vi "rsidr_core_global.vi"() -> ()   [LabVIEW 2020, in "Rohde&Schwarz RTx Oscilloscopes.lvlib"] (continued)
modulation.\n\nAvailable Repeated Capabilities:\nNone\n\nRemote-control command(s):\nWGENerator:MODulation:ASK:FREQuency"}, {"Level"=5, "Class Only"=FALSE, "Identifier"="RSRTX_ATTR_WAVEFORM_GENERATOR_ASK_MODULATION_DEPTH", "Descriptive Name"="Waveform Generator ASK Modulation Depth", "Data Type"=1, "Command"="WGEN:MOD:ASK:DEPT", "Access"=2, "Range Table"="", "Read Callback"="", "Write Callback"="", "Supported Models"="", "Instrument Options"="", "Flags"=0, "Help"="Sets the ASK modulation depth.\n\nAvailable Repeated Capabilities:\nNone\n\nRemote-control command(s):\nWGENerator:MODulation:ASK:DEPTh"}, {"Level"=4, "Class Only"=TRUE, "Identifier"="", "Descriptive Name"="FSK", "Data Type"=0, "Command"="", "Access"=0, "Range Table"="", "Read Callback"="", "Write Callback"="", "Supported Models"="", "Instrument Options"="", "Flags"=0, "Help"="For frequency shift keying (FSK) modulation, the signal switches between Frequency 1 and Frequency 2 at a Hop rate."}, {"Level"=5, "Class Only"=FALSE, "Identifier"="RSRTX_ATTR_WAVEFORM_GENERATOR_FSK_MODULATION_HOPPING_FREQUENCY", "Descriptive Name"="Waveform Generator FSK Modulation Hopping Frequency", "Data Type"=1, "Command"="WGEN:MOD:FSK:HFRE", "Access"=2, "Range Table"="", "Read Callback"="", "Write Callback"="", "Supported Models"="", "Instrument Options"="", "Flags"=0, "Help"="Sets the hopping frequency.\n\nAvailable Repeated Capabilities:\nNone\n\nRemote-control command(s):\nWGENerator:MODulation:FSK:HFREquency"}, {"Level"=5, "Class Only"=FALSE, "Identifier"="RSRTX_ATTR_WAVEFORM_GENERATOR_FSK_MODULATION_RATE", "Descriptive Name"="Waveform Generator FSK Modulation Rate", "Data Type"=1, "Command"="WGEN:MOD:FSK:RATE", "Access"=2, "Range Table"="", "Read Callback"="", "Write Callback"="", "Supported Models"="", "Instrument Options"="", "Flags"=0, "Help"="Sets the hop rate, the time before a switch from the carrier frequency and the modulation frequency.\n\nAvailable Repeated Capabilities:\nNone\n\nRemote-control command(s):\nWGENerator:MODulation:FSK:RATE"}, {"Level"=3, "Class Only"=TRUE, "Identifier"="", "Descriptive Name"="Sweep", "Data Type"=0, "Command"="", "Access"=0, "Range Table"="", "Read Callback"="", "Write Callback"="", "Supported Models"="", "Instrument Options"="", "Flags"=0, "Help"="In the sweep mode, the R&S RTO generates a signal whose frequency gradually changes from the Start frequency to the Stop freuqency for a certain Sweep time."}, {"Level"=4, "Class Only"=FALSE, "Identifier"="RSRTX_ATTR_WAVEFORM_GENERATOR_SWEEP_ENABLED", "Descriptive Name"="Waveform Generator Sweep Enabled", "Data Type"=3, "Command"="WGEN:SWE", "Access"=2, "Range Table"="", "Read Callback"="", "Write Callback"="", "Supported Models"="", "Instrument Options"="", "Flags"=0, "Help"="Enables the sweep.\n\nAvailable Repeated Capabilities:\nNone\n\nRemote-control command(s):\nWGENerator:SWEep[:ENABle]"}, {"Level"=4, "Class Only"=FALSE, "Identifier"="RSRTX_ATTR_WAVEFORM_GENERATOR_SWEEP_TYPE", "Descriptive Name"="Waveform Generator Sweep Type", "Data Type"=0, "Command"="WGEN:SWE:TYPE", "Access"=2, "Range Table"="rsrtx_rngWaveformGeneratorSweepType", "Read Callback"="", "Write Callback"="", "Supported Models"="", "Instrument Options"="", "Flags"=0, "Help"="Configures the sweep type.\n\nAvailable Repeated Capabilities:\nNone\n\nRemote-control command(s):\nWGENerator:SWEep:TYPE"}, {"Level"=4, "Class Only"=FALSE, "Identifier"="RSRTX_ATTR_WAVEFORM_GENERATOR_SWEEP_START_FREQUENCY", "Descriptive Name"="Waveform Generator Sweep Start Frequency", "Data Type"=1, "Command"="WGEN:SWE:FST", "Access"=2, "Range Table"="", "Read Callback"="", "Write Callback"="", "Supported Models"="", "Instrument Options"="", "Flags"=0, "Help"="Sets the start frequency of the sweep range.\n\nAvailable Repeated Capabilities:\nNone\n\nRemote-control command(s):\nWGENerator:SWEep:FSTart"}, {"Level"=4, "Class Only"=FALSE, "Identifier"="RSRTX_ATTR_WAVEFORM_GENERATOR_SWEEP_STOP_FREQUENCY", "Descriptive Name"="Waveform Generator Sweep Stop Frequency", "Data Type"=1, "Command"="WGEN:SWE:FEND", "Access"=2, "Range Table"="", "Read Callback"="", "Write Callback"="", "Supported Models"="", "Instrument Options"="", "Flags"=0, "Help"="Sets the stop frequency of the sweep range.\n\nAvailable Repeated Capabilities:\nNone\n\nRemote-control command(s):\nWGENerator:SWEep:FEND"}, {"Level"=4, "Class Only"=FALSE, "Identifier"="RSRTX_ATTR_WAVEFORM_GENERATOR_SWEEP_TIME", "Descriptive Name"="Waveform Generator Sweep Time", "Data Type"=1, "Command"="WGEN:SWE:TIME", "Access"=2, "Range Table"="", "Read Callback"="", "Write Callback"="", "Supported Models"="", "Instrument Options"="", "Flags"=0, "Help"="Sets the duration of the sweep.\n\nAvailable Repeated Capabilities:\nNone\n\nRemote-control command(s):\nWGENerator:SWEep:TIME"}, {"Level"=3, "Class Only"=TRUE, "Identifier"="", "Descriptive Name"="Arbitrary", "Data Type"=0, "Command"="", "Access"=0, "Range Table"="", "Read Callback"="", "Write Callback"="", "Supported Models"="", "Instrument Options"="", "Flags"=0, "Help"="The arbitrary waveform generator allows you to output a user-defined waveform for testing your devices. You can output a waveform from a file or from the current R&S RTO reference curve format. Files in *.csv and *.bin formats are supported. This files must follow a defined structure."}, {"Level"=4, "Class Only"=FALSE, "Identifier"="RSRTX_ATTR_WAVEFORM_GENERATOR_ARBITRARY_FILE_NAME", "Descriptive Name"="Waveform Generator Arbitrary File Name", "Data Type"=2, "Command"="WGEN:ARB:NAME", "Access"=2, "Range Table"="", "Read Callback"="", "Write Callback"="", "Supported Models"="", "Instrument Options"="", "Flags"=0, "Help"="Sets the file path and the file for an arbitrary waveform.\n\nAvailable Repeated Capabilities:\nNone\n\nRemote-control command(s):\nWGENerator:ARBitrary[:FILE]:NAME"}, {"Level"=4, "Class Only"=FALSE, "Identifier"="RSRTX_ATTR_WAVEFORM_GENERATOR_ARBITRARY_OPEN_FILE", "Descriptive Name"="Waveform Generator Arbitrary Open File", "Data Type"=4, "Command"="WGEN:ARB:OPEN", "Access"=1, "Range Table"="", "Read Callback"="", "Write Callback"="", "Supported Models"="", "Instrument Options"="", "Flags"=0, "Help"="Loads the arbitrary waveform.\n\nAvailable Repeated Capabilities:\nNone\n\nRemote-control command(s):\nWGENerator:ARBitrary[:FILE]:OPEN"}, {"Level"=4, "Class Only"=FALSE, "Identifier"="RSRTX_ATTR_WAVEFORM_GENERATOR_ARBITRARY_SOURCE", "Descriptive Name"="Waveform Generator Arbitrary Source", "Data Type"=0, "Command"="WGEN:ARB:SOUR", "Access"=2, "Range Table"="RsRtx_rngWaveformGeneratorArbitrarySource", "Read Callback"="", "Write Callback"="", "Supported Models"="", "Instrument Options"="", "Flags"=0, "Help"="Selects the oscilloscope source, from which the arbitrary signal is loaded.\n\nAvailable Repeated Capabilities:\nNone\n\nRemote-control command(s):\nWGENerator:ARBitrary:SOURce"}, {"Level"=4, "Class Only"=FALSE, "Identifier"="RSRTX_ATTR_WAVEFORM_GENERATOR_ARBITRARY_UPDATE", "Descriptive Name"="Waveform Generator Arbitrary Update", "Data Type"=4, "Command"="WGEN:ARB:UPD", "Access"=1, "Range Table"="", "Read Callback"="", "Write Callback"="", "Supported Models"="", "Instrument Options"="", "Flags"=0, "Help"="Loads the waveform from the selected signal source.\n\nAvailable Repeated Capabilities:\nNone\n\nRemote-control command(s):\nWGENerator:ARBitrary:UPDate"}, {"Level"=4, "Class Only"=FALSE, "Identifier"="RSRTX_ATTR_WAVEFORM_GENERATOR_ARBITRARY_RANGE_START", "Descriptive Name"="Waveform Generator Arbitrary Range Start", "Data Type"=1, "Command"="WGEN:ARB:RANG:START", "Access"=2, "Range Table"="", "Read Callback"="", "Write Callback"="", "Supported Models"="", "Instrument Options"="", "Flags"=0, "Help"="Sets the start time of the copied waveform part in seconds.\n\nAvailable Repeated Capabilities:\nNone\n\nRemote-control command(s):\nWGENerator:ARBitrary:RANGe:START"}, {"Level"=4, "Class Only"=FALSE, "Identifier"="RSRTX_ATTR_WAVEFORM_GENERATOR_ARBITRARY_RANGE_END", "Descriptive Name"="Waveform Generator Arbitrary Range End", "Data Type"=1, "Command"="WGEN:ARB:RANG:STOP", "Access"=2, "Range Table"="", "Read Callback"="", "Write Callback"="", "Supported Models"="", "Instrument Options"="", "Flags"=0, "Help"="Sets the end time of the copied waveform part in seconds.\n\nAvailable Repeated Capabilities:\nNone\n\nRemote-control command(s):\nWGENerator:ARBitrary:RANGe:STOP"}, {"Level"=4, "Class Only"=FALSE, "Identifier"="RSRTX_ATTR_WAVEFORM_GENERATOR_ARBITRARY_DISPLAY_ENABLE", "Descriptive Name"="Waveform Generator Arbitrary Display Enable", "Data Type"=3, "Command"="WGEN:ARB:VIS", "Access"=2, "Range Table"="", "Read Callback"="", "Write Callback"="", "Supported Models"="", "Instrument Options"="", "Flags"=0, "Help"="Enables the display of the arbitrary waveform.\n\nAvailable Repeated Capabilities:\nNone\n\nRemote-control command(s):\nWGENerator:ARBitrary:VISible"}, {"Level"=3, "Class Only"=TRUE, "Identifier"="", "Descriptive Name"="Output", "Data Type"=0, "Command"="", "Access"=0, "Range Table"="", "Read Callback"="", "Write Callback"="", "Supported Models"="", "Instrument Options"="", "Flags"=0, "Help"="Configures the output values of generator."}, {"Level"=4, "Class Only"=FALSE, "Identifier"="RSRTX_ATTR_WAVEFORM_GENERATOR_OUTPUT_ENABLED", "Descriptive Name"="Waveform Generator Output Enabled", "Data Type"=3, "Command"="WGEN:OUTP", "Access"=2, "Range Table"="", "Read Callback"="", "Write Callback"="", "Supported Models"="", "Instrument Options"="", "Flags"=0, "Help"="Enables the waveform generator and outputs the waveform.\n\nAvailable Repeated Capabilities:\nNone\n\nRemote-control command(s):\nWGENerator:OUTPut[:ENABle]"}, {"Level"=4, "Class Only"=FALSE, "Identifier"="RSRTX_ATTR_WAVEFORM_GENERATOR_OUTPUT_AMPLITUDE", "Descriptive Name"="Waveform Generator Output Amplitude", "Data Type"=1, "Command"="WGEN:VOLT", "Access"=2, "Range Table"="", "Read Callback"="", "Write Callback"="", "Supported Models"="", "Instrument Options"="", "Flags"=0, "Help"="Sets the amplitude, peak to peak voltage, of the output waveform. This is defined as the voltage difference between the maximum and the minimum voltage levels.\n\nAvailable Repeated Capabilities:\nNone\n\nRemote-control command(s):\nWGENerator:VOLTage"}, {"Level"=4, "Class Only"=FALSE, "Identifier"="RSRTX_ATTR_WAVEFORM_GENERATOR_OUTPUT_OFFSET", "Descriptive Name"="Waveform Generator Output Offset", "Data Type"=1, "Command"="WGEN:VOLT:OFFS", "Access"=2, "Range Table"="", "Read Callback"="", "Write Callback"="", "Supported Models"="", "Instrument Options"="", "Flags"=0, "Help"="Sets a voltage offset.\n\nAvailable Repeated Capabilities:\nNone\n\nRemote-control command(s):\nWGENerator:VOLTage:OFFSet"}, {"Level"=4, "Class Only"=FALSE, "Identifier"="RSRTX_ATTR_WAVEFORM_GENERATOR_OUTPUT_USER_LOAD", "Descriptive Name"="Waveform Generator Output User Load", "Data Type"=0, "Command"="WGEN:OUTP:LOAD", "Access"=2, "Range Table"="RsRtx_rngWaveformGeneratorLoad", "Read Callback"="", "Write Callback"="", "Supported Models"="", "Instrument Options"="", "Flags"=0, "Help"="Sets the load of the DUT at its connection.\n\nAvailable Repeated Capabilities:\nNone\n\nRemote-control command(s):\nWGENerator:OUTPut:LOAD"}, {"Level"=4, "Class Only"=FALSE, "Identifier"="RSRTX_ATTR_WAVEFORM_GENERATOR_OUTPUT_DESTINATION", "Descriptive Name"="Waveform Generator Output Destination", "Data Type"=0, "Command"="WGEN:OUTP:DEST", "Access"=2, "Range Table"="RsRtx_rngWaveformGeneratorOutputDestination", "Read Callback"="", "Write Callback"="", "Supported Models"="", "Instrument Options"="", "Flags"=0, "Help"="Configures the output destination.\n\nAvailable Repeated Capabilities:\nNone\n\nRemote-control command(s):\nWGENerator:OUTPut:DESTination"}, {"Level"=3, "Class Only"=TRUE, "Identifier"="", "Descriptive Name"="Noise", "Data Type"=0, "Command"="", "Access"=0, "Range Table"="", "Read Callback"="", "Write Callback"="", "Supported Models"="", "Instrument Options"="", "Flags"=0, "Help"="Configures the noise of attributes."}, {"Level"=4, "Class Only"=FALSE, "Identifier"="RSRTX_ATTR_WAVEFORM_GENERATOR_NOISE_LEVEL_PERCENT", "Descriptive Name"="Waveform Generator Noise Level Percent", "Data Type"=1, "Command"="WGEN:NOIS:REL", "Access"=2, "Range Table"="RsRtx_rngPercent", "Read Callback"="", "Write Callback"="", "Supported Models"="", "Instrument Options"="", "Flags"=0, "Help"="Sets the noise level in percentage of the amplitude.\n\nAvailable Repeated Capabilities:\nNone\n\nRemote-control command(s):\nWGENerator:NOISe:RELative"}, {"Level"=4, "Class Only"=FALSE, "Identifier"="RSRTX_ATTR_WAVEFORM_GENERATOR_NOISE_ABSOLUTE_LEVEL", "Descriptive Name"="Waveform Generator Noise Absolute Level", "Data Type"=1, "Command"="WGEN:NOIS:ABS", "Access"=2, "Range Table"="", "Read Callback"="", "Write Callback"="", "Supported Models"="", "Instrument Options"="", "Flags"=0, "Help"="Sets the level of the noise in volts.\n\nAvailable Repeated Capabilities:\nNone\n\nRemote-control command(s):\nWGENerator:NOISe:ABSolute"}, {"Level"=3, "Class Only"=TRUE, "Identifier"="", "Descriptive Name"="Burst", "Data Type"=0, "Command"="", "Access"=0, "Range Table"="", "Read Callback"="", "Write Callback"="", "Supported Models"="", "Instrument Options"="", "Flags"=0, "Help"="This class contains settings for the waveform generator burst mode. With the burst mode, you can output a waveform for a set number of times."}, {"Level"=4, "Class Only"=FALSE, "Identifier"="RSRTX_ATTR_WAVEFORM_GENERATOR_BURST_ENABLE", "Descriptive Name"="Waveform Generator Burst Enable", "Data Type"=3, "Command"="WGEN:BURS", "Access"=2, "Range Table"="", "Read Callback"="", "Write Callback"="", "Supported Models"="", "Instrument Options"="", "Flags"=0, "Help"="Enables or disables the burst for the generator.\n\nAvailable Repeated Capabilities:\nNone\n\nRemote-control command(s):\nWGENerator:BURSt[:STATe]"}, {"Level"=4, "Class Only"=FALSE, "Identifier"="RSRTX_ATTR_WAVEFORM_GENERATOR_BURST_CYCLES", "Descriptive Name"="Waveform Generator Burst Cycles", "Data Type"=0, "Command"="WGEN:BURS:NCYC", "Access"=2, "Range Table"="RsRtx_rngBurstCycles", "Read Callback"="", "Write Callback"="", "Supported Models"="", "Instrument Options"="", "Flags"=0, "Help"="Sets the number of times the generator outputs one cycle of the waveform per burst.\n\nAvailable Repeated Capabilities:\nNone\n\nRemote-control command(s):\nWGENerator:BURSt:NCYCle"}, {"Level"=4, "Class Only"=FALSE, "Identifier"="RSRTX_ATTR_WAVEFORM_GENERATOR_BURST_IDLE_TIME", "Descriptive Name"="Waveform Generator Burst Idle Time", "Data Type"=1, "Command"="WGEN:BURS:ITIM", "Access"=2, "Range Table"="RsRtx_rngBurstIdleTime", "Read Callback"="", "Write Callback"="", "Supported Models"="", "Instrument Options"="", "Flags"=0, "Help"="Sets the idle time between two burst cycles.\n\nAvailable Repeated Capabilities:\nNone\n\nRemote-control command(s):\nWGENerator:BURSt:ITIMe"}, {"Level"=4, "Class Only"=FALSE, "Identifier"="RSRTX_ATTR_WAVEFORM_GENERATOR_BURST_PHASE_OFFSET", "Descriptive Name"="Waveform Generator Burst Phase Offset", "Data Type"=1, "Command"="WGEN:BURS:PHAS", "Access"=2, "Range Table"="RsRtx_rng360Degrees", "Read Callback"="", "Write Callback"="", "Supported Models"="", "Instrument Options"="", "Flags"=0, "Help"="Sets the start phase of the burst.\n\nAvailable Repeated Capabilities:\nNone\n\nRemote-control command(s):\nWGENerator:BURSt:PHASe"}, {"Level"=4, "Class Only"=FALSE, "Identifier"="RSRTX_ATTR_WAVEFORM_GENERATOR_BURST_TRIGGER_MODE", "Descriptive Name"="Waveform Generator Burst Trigger Mode", "Data Type"=0, "Command"="WGEN:BURS:TRIG", "Access"=2, "Range Table"="RsRtx_rngBurstTriggerMode", "Read Callback"="", "Write Callback"="", "Supported Models"="", "Instrument Options"="", "Flags"=0, "Help"="Selects the trigger mode. Each time the generator receives a trigger, it outputs a burst with the number of cycles defined with RSRTX_ATTR_WAVEFORM_GENERATOR_BURST_CYCLES.\n\nAvailable Repeated Capabilities:\nNone\n\nRemote-control command(s):\nWGENerator:BURSt:TRIGger[:MODE]"}, {"Level"=4, "Class Only"=FALSE, "Identifier"="RSRTX_ATTR_WAVEFORM_GENERATOR_BURST_TRIGGER_SINGLE", "Descriptive Name"="Waveform Generator Burst Trigger Single", "Data Type"=4, "Command"="WGEN:BURS:TRIG:SING", "Access"=1, "Range Table"="", "Read Callback"="", "Write Callback"="", "Supported Models"="", "Instrument Options"="", "Flags"=0, "Help"="Outputs one burst if RSRTX_ATTR_WAVEFORM_GENERATOR_BURST_TRIGGER_MODE is set to Single.\n\nAvailable Repeated Capabilities:\nNone\n\nRemote-control command(s):\nWGENerator:BURSt:TRIGger:SINGle"}, {"Level"=2, "Class Only"=TRUE, "Identifier"="", "Descriptive Name"="Pattern Generator", "Data Type"=0, "Command"="", "Access"=0, "Range Table"="", "Read Callback"="", "Write Callback"="", "Supported Models"="", "Instrument Options"="", "Flags"=0, "Help"="Includes an integrated pattern generator which can generate patterns during testing."}, {"Level"=3, "Class Only"=FALSE, "Identifier"="RSRTX_ATTR_PATTERN_GENERATOR_ENABLED", "Descriptive Name"="Pattern Generator Enabled", "Data Type"=3, "Command"="PGEN:PATT:STAT", "Access"=2, "Range Table"="", "Read Callback"="", "Write Callback"="", "Supported Models"="", "Instrument Options"="", "Flags"=0, "Help"="Enables the pattern generator and outputs the waveform.\n\nAvailable Repeated Capabilities:\nNone\n\nRemote-control command(s):\nPGENerator:PATTern:STATe"}, {"Level"=3, "Class Only"=FALSE, "Identifier"="RSRTX_ATTR_PATTERN_GENERATOR_FUNCTION_TYPE", "Descriptive Name"="Pattern Generator Function Type", "Data Type"=0, "Command"="PGEN:FUNC", "Access"=2, "Range Table"="RsRtx_rngPatternGeneratorFunctionType", "Read Callback"="", "Write Callback"="", "Supported Models"="", "Instrument Options"="", "Flags"=0, "Help"="Selects the pattern generator function.\n\nAvailable Repeated Capabilities:\nNone\n\nRemote-control command(s):\nPGENerator:FUNCtion"}, {"Level"=3, "Class Only"=FALSE, "Identifier"="RSRTX_ATTR_PATTERN_GENERATOR_FREQUENCY", "Descriptive Name"="Pattern Generator Frequency", "Data Type"=1, "Command"="PGEN:PATT:FREQ", "Access"=2, "Range Table"="", "Read Callback"="", "Write Callback"="", "Supported Models"="", "Instrument Options"="", "Flags"=0, "Help"="Configures generator frequency.\n\nAvailable Repeated Capabilities:\nNone\n\nRemote-control command(s):\nPGENerator:PATTern:FREQuency"}, {"Level"=3, "Class Only"=FALSE, "Identifier"="RSRTX_ATTR_PATTERN_GENERATOR_PERIOD", "Descriptive Name"="Pattern Generator Period", "Data Type"=1, "Command"="PGEN:PATT:PER", "Access"=2, "Range Table"="", "Read Callback"="", "Write Callback"="", "Supported Models"="", "Instrument Options"="", "Flags"=0, "Help"="Configures pattern generator period.\n\nAvailable Repeated Capabilities:\nNone\n\nRemote-control command(s):\nPGENerator:PATTern:PERiod"}, {"Level"=3, "Class Only"=FALSE, "Identifier"="RSRTX_ATTR_PATTERN_GENERATOR_POLARITY", "Descriptive Name"="Pattern Generator Polarity", "Data Type"=0, "Command"="PGEN:PATT:SQU:POL", "Access"=2, "Range Table"="rsrtx_rngChannelPolarity", "Read Callback"="", "Write Callback"="", "Supported Models"="", "Instrument Options"="", "Flags"=0, "Help"="Configures the waveform polarity.\n\nAvailable Repeated Capabilities:\nNone\n\nRemote-control command(s):\nPGENerator:PATTern:SQUarewave:POLarity"}, {"Level"=3, "Class Only"=FALSE, "Identifier"="RSRTX_ATTR_PATTERN_GENERATOR_OUTPUT_VOLTAGE", "Descriptive Name"="Pattern Generator Output Voltage", "Data Type"=1, "Command"="PGEN:OUTP:VOLT", "Access"=2, "Range Table"="", "Read Callback"="", "Write Callback"="", "Supported Models"="", "Instrument Options"="", "Flags"=0, "Help"="Sets the output voltage of the generated pattern signal.\n\nAvailable Repeated Capabilities:\nNone\n\nRemote-control command(s):\nPGENerator:OUTPut:VOLTage"}, {"Level"=3, "Class Only"=FALSE, "Identifier"="RSRTX_ATTR_PATTERN_GENERATOR_DUTY_CYCLE", "Descriptive Name"="Pattern Generator Duty Cycle", "Data Type"=1, "Command"="PGEN:PATT:SQU:DCYC", "Access"=2, "Range Table"="", "Read Callback"="", "Write Callback"="", "Supported Models"="", "Instrument Options"="", "Flags"=0, "Help"="Configures the waveform duty cycle.\n\nAvailable Repeated Capabilities:\nNone\n\nRemote-control command(s):\nPGENerator:PATTern:SQUarewave:DCYCle"}, {"Level"=3, "Class Only"=FALSE, "Identifier"="RSRTX_ATTR_PATTERN_GENERATOR_SAMPLE_TIME", "Descriptive Name"="Pattern Generator Sample Time", "Data Type"=1, "Command"="PGEN:PATT:STIM", "Access"=2, "Range Table"="", "Read Callback"="", "Write Callback"="", "Supported Models"="", "Instrument Options"="", "Flags"=0, "Help"="Configures generator sample time.\n\nAvailable Repeated Capabilities:\nNone\n\nRemote-control command(s):\nPGENerator:PATTern:STIMe"}, {"Level"=3, "Class Only"=FALSE, "Identifier"="RSRTX_ATTR_PATTERN_GENERATOR_COUNTER_DIRECTION", "Descriptive Name"="Pattern Generator Counter Direction", "Data Type"=0, "Command"="PGEN:PATT:COUN:DIR", "Access"=2, "Range Table"="RsRtx_rngPatternGeneratorCounterDirection", "Read Callback"="", "Write Callback"="", "Supported Models"="", "Instrument Options"="", "Flags"=0, "Help"="Configures the counter direction.\n\nAvailable Repeated Capabilities:\nNone\n\nRemote-control command(s):\nPGENerator:PATTern:COUNter:DIRection"}, {"Level"=3, "Class Only"=FALSE, "Identifier"="RSRTX_ATTR_PATTERN_GENERATOR_COUNTER_FREQUENCY", "Descriptive Name"="Pattern Generator Counter Frequency", "Data Type"=1, "Command"="PGEN:PATT:COUN:FREQ", "Access"=2, "Range Table"="", "Read Callback"="", "Write Callback"="", "Supported Models"="", "Instrument Options"="", "Flags"=0, "Help"="Defines the frequency value of the pattern generator counter function. The user frequency always refers to the switching of the pattern condition. This results in square waveforms for individual pins.\n\nPin: Frequency\nS0: f/2\nS1: f/4\nS2: f/8\nS3: f/16\n\nAvailable Repeated Capabilities:\nNone\n\nRemote-control command(s):\nPGENerator:PATTern:COUNter:FREQuency"}, {"Level"=3, "Class Only"=FALSE, "Identifier"="RSRTX_ATTR_PATTERN_GENERATOR_BURST_ENABLED", "Descriptive Name"="Pattern Generator Burst Enabled", "Data Type"=3, "Command"="PGEN:PATT:BURS:STAT", "Access"=2, "Range Table"="", "Read Callback"="", "Write Callback"="", "Supported Models"="", "Instrument Options"="", "Flags"=0, "Help"="Turns burst on/off.\n\nAvailable Repeated Capabilities:\nNone\n\nRemote-control command(s):\nPGENerator:PATTern:BURSt:STATe"}, {"Level"=3, "Class Only"=FALSE, "Identifier"="RSRTX_ATTR_PATTERN_GENERATOR_BURST_CYCLES", "Descriptive Name"="Pattern Generator Burst Cycles", "Data Type"=0, "Command"="PGEN:PATT:BURS:NCYC", "Access"=2, "Range Table"="", "Read Callback"="", "Write Callback"="", "Supported Models"="", "Instrument Options"="", "Flags"=0, "Help"="Configures number of burst cycles.\n\nAvailable Repeated Capabilities:\nNone\n\nRemote-control command(s):\nPGENerator:PATTern:BURSt:NCYCle"}, {"Level"=3, "Class Only"=FALSE, "Identifier"="RSRTX_ATTR_PATTERN_GENERATOR_IDLE_TIME", "Descriptive Name"="Pattern Generator Idle Time", "Data Type"=1, "Command"="PGEN:PATT:ITIM", "Access"=2, "Range Table"="", "Read Callback"="", "Write Callback"="", "Supported Models"="", "Instrument Options"="", "Flags"=0, "Help"="Configures generator idle time.\n\nAvailable Repeated Capabilities:\nNone\n\nRemote-control command(s):\nPGENerator:PATTern:ITIMe"}, {"Level"=3, "Class Only"=FALSE, "Identifier"="RSRTX_ATTR_PATTERN_GENERATOR_TRIGGER_MODE", "Descriptive Name"="Pattern Generator Trigger Mode", "Data Type"=0, "Command"="PGEN:PATT:TRIG:MODE", "Access"=2, "Range Table"="RsRtx_rngPatternGeneratorTriggerMode", "Read Callback"="", "Write Callback"="", "Supported Models"="", "Instrument Options"="", "Flags"=0, "Help"="Configures the trigger mode.\n\nAvailable Repeated Capabilities:\nNone\n\nRemote-control command(s):\nPGENerator:PATTern:TRIGger:MODE"}, {"Level"=3, "Class Only"=FALSE, "Identifier"="RSRTX_ATTR_PATTERN_GENERATOR_TRIGGER_RUN_SINGLE", "Descriptive Name"="Pattern Generator Trigger Run Single", "Data Type"=4, "Command"="PGEN:PATT:TRIG:SING", "Access"=1, "Range Table"="", "Read Callback"="", "Write Callback"="", "Supported Models"="", "Instrument Options"="", "Flags"=0, "Help"="Run pattern trigur once.\n\nAvailable Repeated Capabilities:\nNone\n\nRemote-control command(s):\nPGENerator:PATTern:TRIGger:SINGle"}, {"Level"=3, "Class Only"=FALSE, "Identifier"="RSRTX_ATTR_PATTERN_GENERATOR_EXTERNAL_TRIGGER_SLOPE", "Descriptive Name"="Pattern Generator External Trigger Slope", "Data Type"=0, "Command"="PGEN:PATT:TRIG:EXT:SLOP", "Access"=2, "Range Table"="rsrtx_rngTriggerSlope", "Read Callback"="", "Write Callback"="", "Supported Models"="", "Instrument Options"="", "Flags"=0, "Help"="Defines the slope of the external arbitrary pattern trigger.\n\nAvailable Repeated Capabilities:\nNone\n\nRemote-control command(s):\nPGENerator:PATTern:TRIGger:EXTern:SLOPe"}, {"Level"=3, "Class Only"=TRUE, "Identifier"="", "Descriptive Name"="ARB", "Data Type"=0, "Command"="", "Access"=0, "Range Table"="", "Read Callback"="", "Write Callback"="", "Supported Models"="", "Instrument Options"="", "Flags"=0, "Help"="Configures ARB waveform."}, {"Level"=4, "Class Only"=FALSE, "Identifier"="RSRTX_ATTR_PATTERN_GENERATOR_ARB_PATTERN_LENGTH", "Descriptive Name"="Pattern Generator ARB Pattern Length", "Data Type"=0, "Command"="PGEN:PATT:ARB:DATA:LENG", "Access"=2, "Range Table"="", "Read Callback"="", "Write Callback"="", "Supported Models"="", "Instrument Options"="", "Flags"=0, "Help"="Configures pattern generator data length.\n\nAvailable Repeated Capabilities:\nNone\n\nRemote-control command(s):\nPGENerator:PATTern:ARBitrary:DATA:LENGth"}, {"Level"=4, "Class Only"=FALSE, "Identifier"="RSRTX_ATTR_PATTERN_GENERATOR_ARB_INDEX", "Descriptive Name"="Pattern Generator ARB Index", "Data Type"=0, "Command"="PGEN:PATT:ARB:DATA:APP:IND", "Access"=2, "Range Table"="", "Read Callback"="", "Write Callback"="", "Supported Models"="", "Instrument Options"="", "Flags"=0, "Help"="Configures the ARB index.\n\nAvailable Repeated Capabilities:\nNone\n\nRemote-control command(s):\nPGENerator:PATTern:ARBitrary:DATA:APPend:INDex"}, {"Level"=3, "Class Only"=TRUE, "Identifier"="", "Descriptive Name"="Manual", "Data Type"=0, "Command"="", "Access"=0, "Range Table"="", "Read Callback"="", "Write Callback"="", "Supported Models"="", "Instrument Options"="", "Flags"=0, "Help"="Configures manual."}, {"Level"=4, "Class Only"=FALSE, "Identifier"="RSRTX_ATTR_PATTERN_GENERATOR_MANUAL_STATE", "Descriptive Name"="Pattern Generator Manual State", "Data Type"=3, "Command"="PGEN:MAN:STAT{OutputPin}", "Access"=2, "Range Table"="", "Read Callback"="", "Write Callback"="", "Supported Models"="", "Instrument Options"="", "Flags"=0, "Help"="Configures manual state.\n\nAvailable Repeated Capabilities:\nOutputPin: P0, P1, P2, P3\r\n\nRemote-control command(s):\nPGENerator:MANual:STATe<s>"}, {"Level"=3, "Class Only"=TRUE, "Identifier"="", "Descriptive Name"="PWM", "Data Type"=0, "Command"="", "Access"=0, "Range Table"="", "Read Callback"="", "Write Callback"="", "Supported Models"="", "Instrument Options"="", "Flags"=0, "Help"="You can use the pattern generator to generate several pulse width modulated (PWM)\nsignals: PWM, PWM - RGB LED, PWM-TestSignals."}, {"Level"=4, "Class Only"=FALSE, "Identifier"="RSRTX_ATTR_PATTERN_GENERATOR_PWM_MOTOR_ENABLE", "Descriptive Name"="Pattern Generator PWM Motor Enable", "Data Type"=3, "Command"="PGEN:PATT:PWM:ENAB", "Access"=2, "Range Table"="", "Read Callback"="", "Write Callback"="", "Supported Models"="", "Instrument Options"="", "Flags"=0, "Help"="Switches the motor on or off if the motor driver uses a dedicated enable signal.\n\nAvailable Repeated Capabilities:\nNone\n\nRemote-control command(s):\nPGENerator:PATTern:PWM:ENABle"}, {"Level"=4, "Class Only"=FALSE, "Identifier"="RSRTX_ATTR_PATTERN_GENERATOR_PWM_MOTOR_DIRECTION", "Descriptive Name"="Pattern Generator PWM Motor Direction", "Data Type"=0, "Command"="PGEN:PATT:PWM:DIR", "Access"=2, "Range Table"="RsRtx_rngPWMMotorDirection", "Read Callback"="", "Write Callback"="", "Supported Models"="", "Instrument Options"="", "Flags"=0, "Help"="Sets the direction of motor rotation.\n\nAvailable Repeated Capabilities:\nNone\n\nRemote-control command(s):\nPGENerator:PATTern:PWM:DIRection"}, {"Level"=4, "Class Only"=FALSE, "Identifier"="RSRTX_ATTR_PATTERN_GENERATOR_PWM_DUTY_CYCLE", "Descriptive Name"="Pattern Generator PWM Duty Cycle", "Data Type"=1, "Command"="PGEN:PATT:PWM:DCYC", "Access"=2, "Range Table"="RsRtx_rngPWMDutyCycle", "Read Callback"="", "Write Callback"="", "Supported Models"="", "Instrument Options"="", "Flags"=0, "Help"="Sets the duty cycle of the PWM signal at P0, and thus the motor speed.\n\nAvailable Repeated Capabilities:\nNone\n\nRemote-control command(s):\nPGENerator:PATTern:PWM:DCYCle"}, {"Level"=4, "Class Only"=FALSE, "Identifier"="RSRTX_ATTR_PATTERN_GENERATOR_PWM_LED_INTENSITY", "Descriptive Name"="Pattern Generator PWM LED Intensity", "Data Type"=1, "Command"="PGEN:PATT:LED:INT", "Access"=2, "Range Table"="RsRtx_rngPWMDutyCycle", "Read Callback"="", "Write Callback"="", "Supported Models"="", "Instrument Options"="", "Flags"=0, "Help"="Sets the duty cycle of the signal at P3, which corresponds to the intensity of the light. You can use this signal if the controller supports separate intensity control.\n\nAvailable Repeated Capabilities:\nNone\n\nRemote-control command(s):\nPGENerator:PATTern:LED:INTens"}, {"Level"=4, "Class Only"=FALSE, "Identifier"="RSRTX_ATTR_PATTERN_GENERATOR_PWM_LED_INTENSITY_BLUE", "Descriptive Name"="Pattern Generator PWM LED Intensity Blue", "Data Type"=1, "Command"="PGEN:PATT:LED:BLUE", "Access"=2, "Range Table"="RsRtx_rngPWMDutyCycle", "Read Callback"="", "Write Callback"="", "Supported Models"="", "Instrument Options"="", "Flags"=0, "Help"="Set the duty cycle of the red, green, and blue colors, which corresponds to the color intensity.\n\nAvailable Repeated Capabilities:\nNone\n\nRemote-control command(s):\nPGENerator:PATTern:LED:BLUE"}, {"Level"=4, "Class Only"=FALSE, "Identifier"="RSRTX_ATTR_PATTERN_GENERATOR_PWM_LED_INTENSITY_GREEN", "Descriptive Name"="Pattern Generator PWM LED Intensity Green", "Data Type"=1, "Command"="PGEN:PATT:LED:GRE", "Access"=2, "Range Table"="RsRtx_rngPWMDutyCycle", "Read Callback"="", "Write Callback"="", "Supported Models"="", "Instrument Options"="", "Flags"=0, "Help"="Set the duty cycle of the red, green, and blue colors, which corresponds to the color intensity.\n\nAvailable Repeated Capabilities:\nNone\n\nRemote-control command(s):\nPGENerator:PATTern:LED:GREen"}, {"Level"=4, "Class Only"=FALSE, "Identifier"="RSRTX_ATTR_PATTERN_GENERATOR_PWM_LED_INTENSITY_RED", "Descriptive Name"="Pattern Generator PWM LED Intensity Red", "Data Type"=1, "Command"="PGEN:PATT:LED:RED", "Access"=2, "Range Table"="RsRtx_rngPWMDutyCycle", "Read Callback"="", "Write Callback"="", "Supported Models"="", "Instrument Options"="", "Flags"=0, "Help"="Set the duty cycle of the red, green, and blue colors, which corresponds to the color intensity.\n\nAvailable Repeated Capabilities:\nNone\n\nRemote-control command(s):\nPGENerator:PATTern:LED:RED"}, {"Level"=1, "Class Only"=TRUE, "Identifier"="", "Descriptive Name"="Display", "Data Type"=0, "Command"="", "Access"=0, "Range Table"="", "Read Callback"="", "Write Callback"="", "Supported Models"="", "Instrument Options"="", "Flags"=0, "Help"="Display settings."}, {"Level"=2, "Class Only"=FALSE, "Identifier"="RSRTX_ATTR_COLOR_AND_BRIGHTNESS", "Descriptive Name"="Color And Brightness", "Data Type"=0, "Command"="DISP:PAL", "Access"=2, "Range Table"="rsrtx_rngColorBrightness", "Read Callback"="", "Write Callback"="", "Supported Models"="", "Instrument Options"="", "Flags"=0, "Help"="Sets the color and brightness of the displayed waveform samples depending on their cumulative occurance.\n\nAvailable Repeated Capabilities:\nNone\n\nRemote-control command(s):\nDISPlay:PALette"}, {"Level"=2, "Class Only"=FALSE, "Identifier"="RSRTX_ATTR_SIGNAL_STYLE", "Descriptive Name"="Signal Style", "Data Type"=0, "Command"="DISP:STYL", "Access"=2, "Range Table"="rsrtx_rngSignalStyle", "Read Callback"="", "Write Callback"="", "Supported Models"="", "Instrument Options"="", "Flags"=0, "Help"="Select the style in which the waveform is displayed.\n\nAvailable Repeated Capabilities:\nNone\n\nRemote-control command(s):\nDISPlay:STYLe"}, {"Level"=2, "Class Only"=FALSE, "Identifier"="RSRTX_ATTR_DIAGRAM_GRID_STYLE", "Descriptive Name"="Diagram Grid Style", "Data Type"=0, "Command"="DISP:GRID:STYL", "Access"=2, "Range Table"="rsrtx_rngGridStyle", "Read Callback"="", "Write Callback"="", "Supported Models"="", "Instrument Options"="", "Flags"=0, "Help"="Defines how the grid is displayed.\n\nAvailable Repeated Capabilities:\nNone\n\nRemote-control command(s):\nDISPlay:GRID:STYLe"}, {"Level"=2, "Class Only"=FALSE, "Identifier"="RSRTX_ATTR_DIAGRAM_ANNOTATION_ENABLED", "Descriptive Name"="Diagram Annotation Enabled", "Data Type"=3, "Command"="DISP:GRID:ANN", "Access"=2, "Range Table"="", "Read Callback"="", "Write Callback"="", "Supported Models"="", "Instrument Options"="", "Flags"=0, "Help"="Enables grid annotation.\n\nAvailable Repeated Capabilities:\nNone\n\nRemote-control command(s):\nDISPlay:GRID:ANNotation[:ENABle]"}, {"Level"=2, "Class Only"=FALSE, "Identifier"="RSRTX_ATTR_DIAGRAM_ANNOTATION_TRACK", "Descriptive Name"="Diagram Annotation Track", "Data Type"=0, "Command"="DISP:GRID:ANN:TRAC", "Access"=2, "Range Table"="", "Read Callback"="", "Write Callback"="", "Supported Models"="", "Instrument Options"="", "Flags"=0, "Help"="Configures diagram annotatiom track.\n\nAvailable Repeated Capabilities:\nNone\n\nRemote-control command(s):\nDISPlay:GRID:ANNotation:TRACk"}, {"Level"=2, "Class Only"=FALSE, "Identifier"="RSRTX_ATTR_WAVEFORM_INTENSITY", "Descriptive Name"="Waveform Intensity", "Data Type"=1, "Command"="DISP:INT:WAV", "Access"=2, "Range Table"="rsrtx_rngPct", "Read Callback"="", "Write Callback"="", "Supported Models"="", "Instrument Options"="", "Flags"=0, "Help"="Defines the strength of the waveform line in the diagram.\n\nAvailable Repeated Capabilities:\nNone\n\nRemote-control command(s):\nDISPlay:INTensity:WAVeform"}, {"Level"=2, "Class Only"=FALSE, "Identifier"="RSRTX_ATTR_BACKGROUND_INTENSITY", "Descriptive Name"="Background Intensity", "Data Type"=1, "Command"="DISP:INT:BACK", "Access"=2, "Range Table"="rsrtx_rngBckLight", "Read Callback"="", "Write Callback"="", "Supported Models"="", "Instrument Options"="", "Flags"=0, "Help"="Defines the intensity of the background lighting of the display.\n\nAvailable Repeated Capabilities:\nNone\n\nRemote-control command(s):\nDISPlay:INTensity:BACKlight"}, {"Level"=2, "Class Only"=FALSE, "Identifier"="RSRTX_ATTR_GRID_INTENSITY", "Descriptive Name"="Grid Intensity", "Data Type"=1, "Command"="DISP:INT:GRID", "Access"=2, "Range Table"="rsrtx_rngPct", "Read Callback"="", "Write Callback"="", "Supported Models"="", "Instrument Options"="", "Flags"=0, "Help"="Defines the intensity of the grid on the screen.\n\nAvailable Repeated Capabilities:\nNone\n\nRemote-control command(s):\nDISPlay:INTensity:GRID"}, {"Level"=2, "Class Only"=FALSE, "Identifier"="RSRTX_ATTR_DISPLAY_LANGUAGE", "Descriptive Name"="Display Language", "Data Type"=0, "Command"="DISP:LANG", "Access"=2, "Range Table"="rsrtx_rngLanguage", "Read Callback"="", "Write Callback"="", "Supported Models"="", "Instrument Options"="", "Flags"=0, "Help"="Sets the language in which the softkey labels, help and other screen information can be displayed. Supported languages are listed in the Specifications data sheet.\n\nAvailable Repeated Capabilities:\nNone\n\nRemote-control command(s):\nDISPlay:LANGuage"}, {"Level"=2, "Class Only"=FALSE, "Identifier"="RSRTX_ATTR_DISPLAY_DATE_AND_TIME", "Descriptive Name"="Display Date And Time", "Data Type"=3, "Command"="DISP:DTIM", "Access"=2, "Range Table"="", "Read Callback"="", "Write Callback"="", "Supported Models"="", "Instrument Options"="", "Flags"=0, "Help"="Switches the date and time display in the upper right corner of the screen on or off.\n\nAvailable Repeated Capabilities:\nNone\n\nRemote-control command(s):\nDISPlay:DTIMe"}, {"Level"=2, "Class Only"=FALSE, "Identifier"="RSRTX_ATTR_DIAGRAM_MODE", "Descriptive Name"="Diagram Mode", "Data Type"=0, "Command"="DISP:MODE", "Access"=2, "Range Table"="rsrtx_rngDiagramMode", "Read Callback"="", "Write Callback"="", "Supported Models"="", "Instrument Options"="", "Flags"=0, "Help"="Sets the diagram mode.\n\nAvailable Repeated Capabilities:\nNone\n\nRemote-control command(s):\nDISPlay:MODE"}, {"Level"=2, "Class Only"=FALSE, "Identifier"="RSRTX_ATTR_DISPLAY_SEND_MESSAGE", "Descriptive Name"="Display Send Message", "Data Type"=2, "Command"="DISP:DIAL:MESS", "Access"=1, "Range Table"="", "Read Callback"="", "Write Callback"="", "Supported Models"="", "Instrument Options"="", "Flags"=0, "Help"="Sends a message text to the instrument and displays it in a message box.\n\nAvailable Repeated Capabilities:\nNone\n\nRemote-control command(s):\nDISPlay:DIALog:MESSage"}, {"Level"=2, "Class Only"=FALSE, "Identifier"="RSRTX_ATTR_DISPLAY_CLOSE_DIALOG", "Descriptive Name"="Display Close Dialog", "Data Type"=4, "Command"="DISP:DIAL:CLOS", "Access"=1, "Range Table"="", "Read Callback"="", "Write Callback"="", "Supported Models"="", "Instrument Options"="", "Flags"=0, "Help"="Closes an open dialog box.\n\nAvailable Repeated Capabilities:\nNone\n\nRemote-control command(s):\nDISPlay:DIALog:CLOSe"}, {"Level"=2, "Class Only"=FALSE, "Identifier"="RSRTX_ATTR_DIALOG_TRANSPARENCY", "Descriptive Name"="Dialog Transparency", "Data Type"=0, "Command"="DISP:DIAL:TRAN", "Access"=2, "Range Table"="RsRtx_rngPctInt", "Read Callback"="", "Write Callback"="", "Supported Models"="", "Instrument Options"="", "Flags"=0, "Help"="Sets the transparency of result boxes that overlay the waveforms, for example, boxes with statistical results or digital voltmeter results.\n\nAvailable Repeated Capabilities:\nNone\n\nRemote-control command(s):\nDISPlay:DIALog:TRANsparency"}, {"Level"=2, "Class Only"=FALSE, "Identifier"="RSRTX_ATTR_DISPLAY_CLEAR_SCREEN", "Descriptive Name"="Display Clear Screen", "Data Type"=4, "Command"="DISP:CLE", "Access"=1, "Range Table"="", "Read Callback"="", "Write Callback"="", "Supported Models"="", "Instrument Options"="", "Flags"=0, "Help"="Clears the display.\n\nAvailable Repeated Capabilities:\nNone\n\nRemote-control command(s):\nDISPlay:CLEar[:SCReen]"}, {"Level"=2, "Class Only"=TRUE, "Identifier"="", "Descriptive Name"="Persistence", "Data Type"=0, "Command"="", "Access"=0, "Range Table"="", "Read Callback"="", "Write Callback"="", "Supported Models"="", "Instrument Options"="", "Flags"=0, "Help"="Contains attributes for persistence settings."}, {"Level"=3, "Class Only"=FALSE, "Identifier"="RSRTX_ATTR_PERSISTENCE_ENABLED", "Descriptive Name"="Persistence Enabled", "Data Type"=3, "Command"="DISP:PERS:STAT", "Access"=2, "Range Table"="", "Read Callback"="", "Write Callback"="", "Supported Models"="", "Instrument Options"="", "Flags"=0, "Help"="If enabled, each new data point in the diagram area remains on the screen for the duration defined using DISPlay:PERSistence:TIME, or as long as DISPlay:PERSistence:INFinite is enabled.\nIf disabled, the signal value is only displayed as long as it actually occurs.\n\nAvailable Repeated Capabilities:\nNone\n\nRemote-control command(s):\nDISPlay:PERSistence[:STATe]"}, {"Level"=3, "Class Only"=FALSE, "Identifier"="RSRTX_ATTR_PERSISTENCE_TYPE", "Descriptive Name"="Persistence Type", "Data Type"=0, "Command"="DISP:PERS:TYPE", "Access"=2, "Range Table"="RsRtx_rngPersistenceType", "Read Callback"="", "Write Callback"="", "Supported Models"="", "Instrument Options"="", "Flags"=0, "Help"="Configures the persistence type.\n\nAvailable Repeated Capabilities:\nNone\n\nRemote-control command(s):\nDISPlay:PERSistence:TYPE"}, {"Level"=3, "Class Only"=FALSE, "Identifier"="RSRTX_ATTR_INFINITE_PERSISTENCE", "Descriptive Name"="Infinite Persistence", "Data Type"=3, "Command"="DISP:PERS:INF", 
